vi "Reset Tag.vi"(7 "Tree In":refnum<class "Tree.lvclass">, 8 "error in (no error)":errorcluster, 9 "New Tag":string, 10 "Original Tag":string, 11 "Tree Data in":refnum<class "Tree Data.lvclass">) -> (0 "error out":errorcluster, 3 "Tree Data out":refnum<class "Tree Data.lvclass">, 5 "Tree Out":refnum<class "Tree.lvclass">)   [LabVIEW 2024, in "Tree Data.lvclass"]
uses:
  Tree Data.lvclass
  Tree/Tree.lvclass
  Tree Data.lvclass/Tree Data.ctl
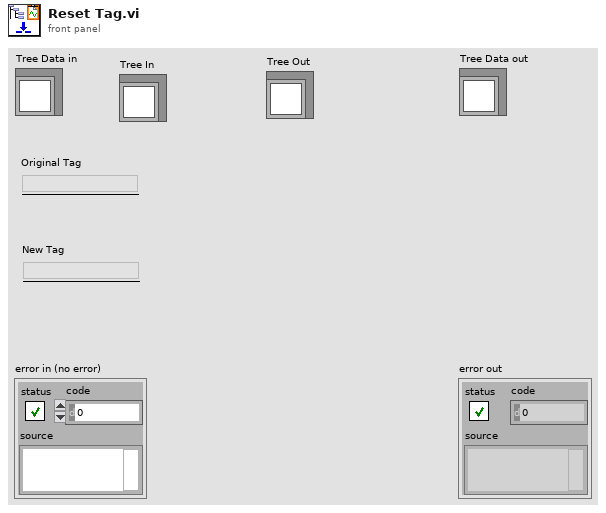
[diagram p1: front panel]
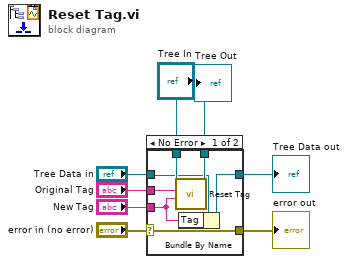
[diagram p0: block diagram]
diagram:
  n1 = case shown="No Error" "error in (no error)" {
    selector: "error in (no error)" -> [w15 w18]
    tunnel: [w15 w18] -> w7
    tunnel: [w9 w17] -> w5
    tunnel: "Tree Data in" -> [w11 w17]
    tunnel: "Tree In" -> [w14 w16]
    tunnel: [w13 w16] -> w3
    tunnel: "Original Tag" -> [w12 _]
    tunnel: "New Tag" -> [w10 _]
    frame No Error {
      n2 = call "Reset Tag.vi"("New Tag"=w10, "Original Tag"=w12, "Tree in"=w14) -> ("Tree out"=w13:refnum<class "Tree.lvclass">)  [unwired: 7 in, 1 out]
      n3 = Bundle By Name(cluster=w11, "Tag"=w10) -> (w9:refnum<class "Tree Data.lvclass">)
    }
    frame Error {
    }
  }
  "error out" <- w7
  "Tree Data out" <- w5
  "Tree Out" <- w3
